vi "Read # holes in one.vi"(8 "error in (no error)":errorcluster, 11 "Golf Player in":refnum<class "Golf Player.lvclass">) -> (0 "error out":errorcluster, 2 "# holes in one":i32, 3 "Golf Player out":refnum<class "Golf Player.lvclass">)   [LabVIEW 2019, in "Golf Player.lvclass"]
uses:
  Golf Player.lvclass
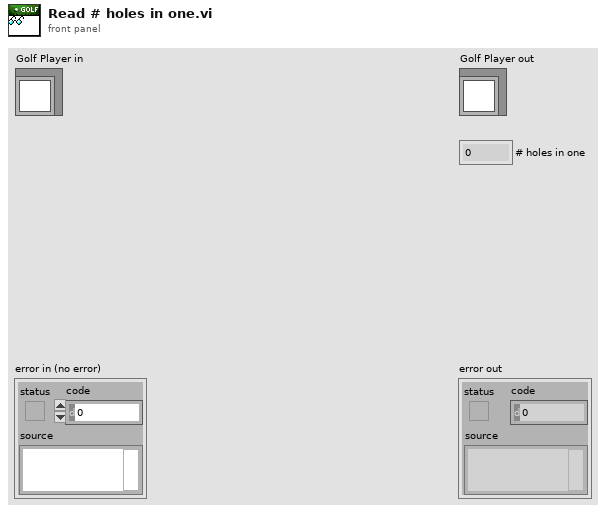
[diagram p1: front panel]
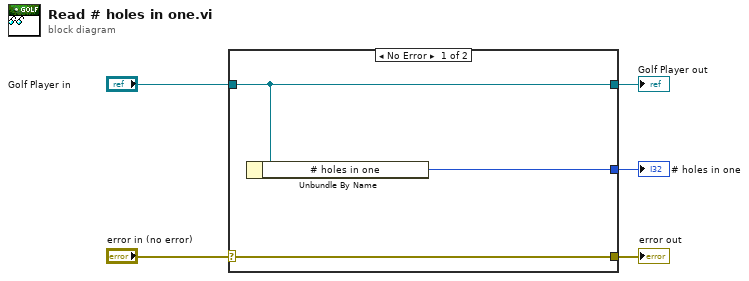
[diagram p0: block diagram]
diagram:
  n1 = case shown="No Error" "error in (no error)" {
    selector: "error in (no error)" -> [w8 w9]
    tunnel: [w8 w9] -> w4
    tunnel: [w7 w10] -> w2
    tunnel: "Golf Player in" -> [w7 w10]
    tunnel: [w6 _] -> w1
    frame No Error {
      n2 = Unbundle By Name(w7) -> ("# holes in one"=w6:i32)
    }
    frame Error {
    }
  }
  "error out" <- w4
  "Golf Player out" <- w2
  "# holes in one" <- w1
